vi "practica1_3.2.vi"() -> ()   [LabVIEW 2016]
panel:
  out "ultimo valor\nde coseno":dbl
  out "maximo":dbl[](array[numeric])
  out "señales seno y coseno":dbl[][](graph)
  # "se muestran las dos señales \nseno en verde y coseno en rojo"
  # "aun que se puedan cambiar los nombres\ny colores de las señales en la parte superior \nsolo muestra la primera"
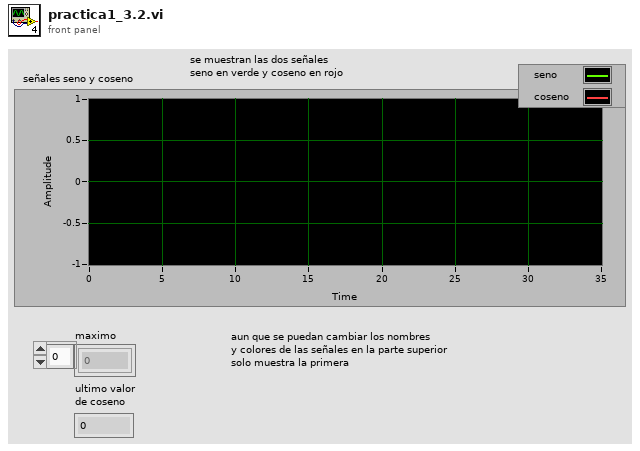
[diagram p1: front panel]
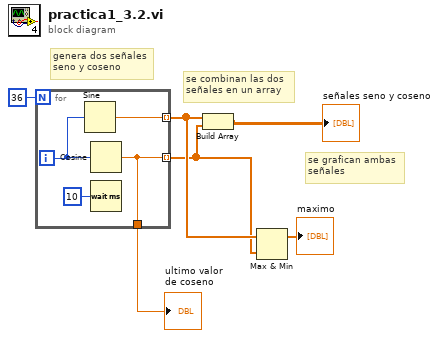
[diagram p0: block diagram]
diagram:
  # "se grafican ambas\nseñales"
  # "se combinan las dos\nseñales en un array"
  # "genera dos señales\nseno y coseno"
  n1 = for {
    N: 36 -> [_]
    tunnel: [w10] -> w4 mode=indexing
    tunnel: [w7] -> w3 mode=indexing
    tunnel: [w7] -> w1
    i -> [w8]
    n2 = Sine(x=w8) -> (sin(x)=w10:dbl)
    n3 = Cosine(x=w8) -> (cos(x)=w7:dbl)
    n4 = Wait (ms)(milliseconds to wait=u32 10) -> ()  [unwired: 1 out]
  }
  "ultimo valor\nde coseno" <- w1
  n5 = Build Array(w4, w3) -> (→"señales seno y coseno":dbl[][])
  n6 = Max & Min(x=w4, y=w3) -> (max(x,y)=→"maximo":dbl[])  [unwired: 1 out]
